vi "Recalculate Servo Position.vi"(10 "Position in Degrees":u16=90, 11 "Serwo Steps Per Turn (48)":u16=48) -> (2 "Recalculated Position":u16, 3 "Recalculated Position string":string)   [LabVIEW 2017]
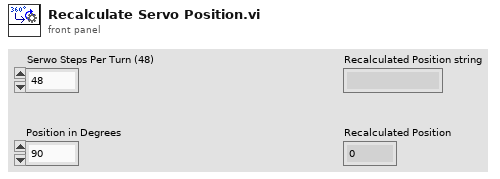
[diagram p1: front panel]
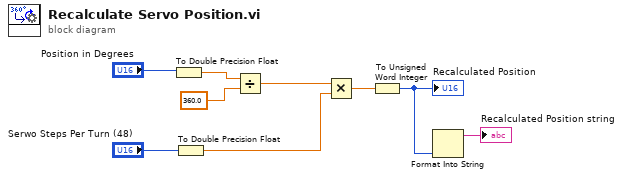
[diagram p0: block diagram]
diagram:
  n1 = To Double Precision Float(number="Position in Degrees") -> (double precision float=w8:dbl)
  n2 = To Double Precision Float(number="Serwo Steps Per Turn (48)") -> (double precision float=w4:dbl)
  n3 = Divide(x=w8, y=360.0) -> (x/y=w6:dbl)
  n4 = Multiply(x=w6, y=w4) -> (x*y=w3:dbl)
  n5 = To Unsigned Word Integer(number=w3) -> (unsigned 16bit integer=w2:u16)
  "Recalculated Position" <- w2
  n6 = Format Into String(w2) -> (resulting string=→"Recalculated Position string":string)  [unwired: 3 in, 1 out]
